vi "TagBus_Read_DELETEME.vi"(10 "Tag Key Array":string[](array[string]), 11 "TagBus.lvclass":refnum<class "TagBus.lvclass">) -> (2 "Value Array":dbl[](array[numeric]), 3 "TagBus.lvclass out":refnum<class "TagBus.lvclass">)   [LabVIEW 2015]
uses:
  TagBus.lvclass
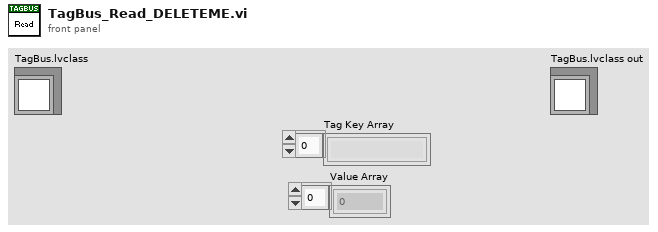
[diagram p1: front panel]
types:
  T1 = typedef "tag bus.lvlib/data table.lvlib/data table.ctl" = cluster{"Double":dbl[], "Single":sgl[], "I64":i64[], "I32":i32[], "I16":i16[], "I8":i8[], "U64":u64[], "U32":u32[], "U16":u16[], "U8":u8[], "Boolean":bool[], "String":string[], "Array of Double":cluster{"DBL Array":dbl[]}[], "Array of Single":cluster{"SGL Array":sgl[]}[], "Array of I64":cluster{"I64 Array":i64[]}[], "Array of I32":cluster{"I32 Array":i32[]}[], "Array of I16":cluster{"I16 Array":i16[]}[], "Array of I8":cluster{"I8 Array":i8[]}[], "Array of U64":cluster{"U64 Array":u64[]}[], "Array of U32":cluster{"U32 Array":u32[]}[], "Array of U16":cluster{"U16 Array":u16[]}[], "Array of U8":cluster{"U8 Array":u8[]}[], "Array of Boolean":cluster{"Boolean Array":bool[]}[], "Array of String":cluster{"String Array":string[]}[]}
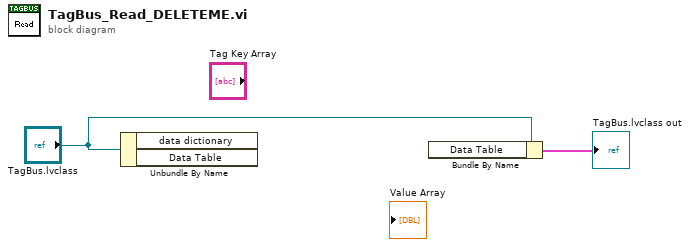
[diagram p0: block diagram]
diagram:
  n1 = Unbundle By Name("TagBus.lvclass") -> ("data dictionary"=w6, "Data Table"=w5)
  n2 = Bundle By Name(cluster="TagBus.lvclass") -> (→"TagBus.lvclass out":cluster{}, "Data Table"=w4:T1)
